vi "泰克1路.vi"() -> ()   [LabVIEW 2018]
uses:
  <instrlib>/Tektronix DPO MSO 2000 4000 Series/Public/Configure/Configure Trigger (Edge).vi
  <vilib>/Utility/file.llb/Write Delimited Spreadsheet (string).vi
  <instrlib>/Tektronix DPO MSO 2000 4000 Series/Tektronix DPO MSO 2000 4000 Series.lvlib
  <vilib>/Utility/file.llb/Write Delimited Spreadsheet (DBL).vi
panel:
  out "波形图表":waveform(dbl)(graph)
  out "Frequency":dbl
  out "rasing":dbl
  out "error out":errorcluster
  in  "停止":bool
  out "num":u32
  in  "VISA Resource Name":refnum<visa-resource-name>="TCPIP::192.168.129.100::INSTR"
  in  "VoltRange-1(V=10*grid)":dbl=0.005
  in  "Trigger Level (V)":dbl=0.01
  in  "Timebase(s)":dbl=4e-08
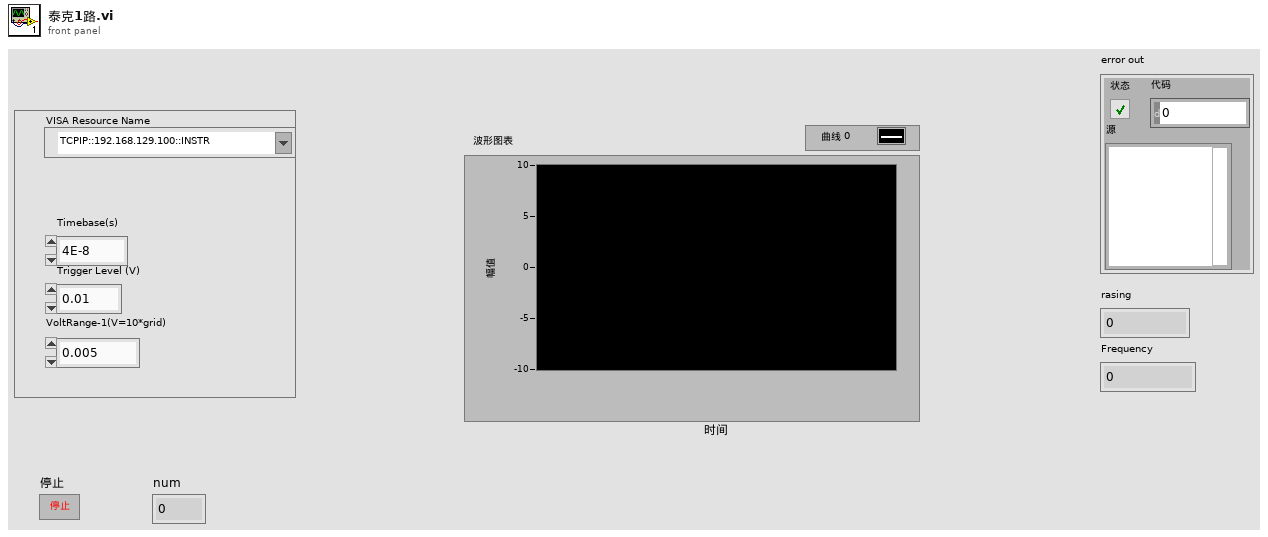
[diagram p1: front panel]
types:
  T1 = enum16{"Channel 1", "Channel 2", "Channel 3", "Channel 4", "Math", "Reference 1", "Reference 2", "Reference 3", "Reference 4"}
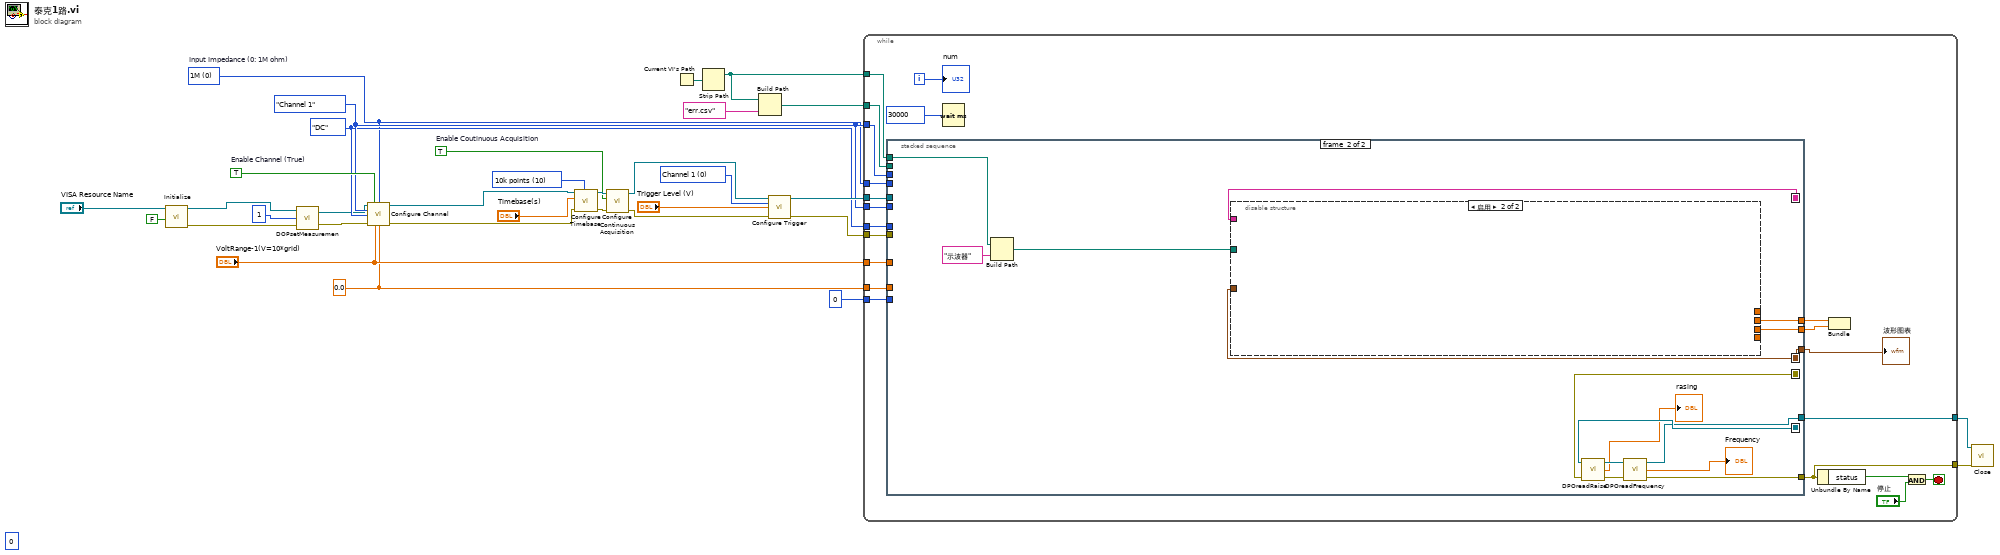
[diagram p0: block diagram]
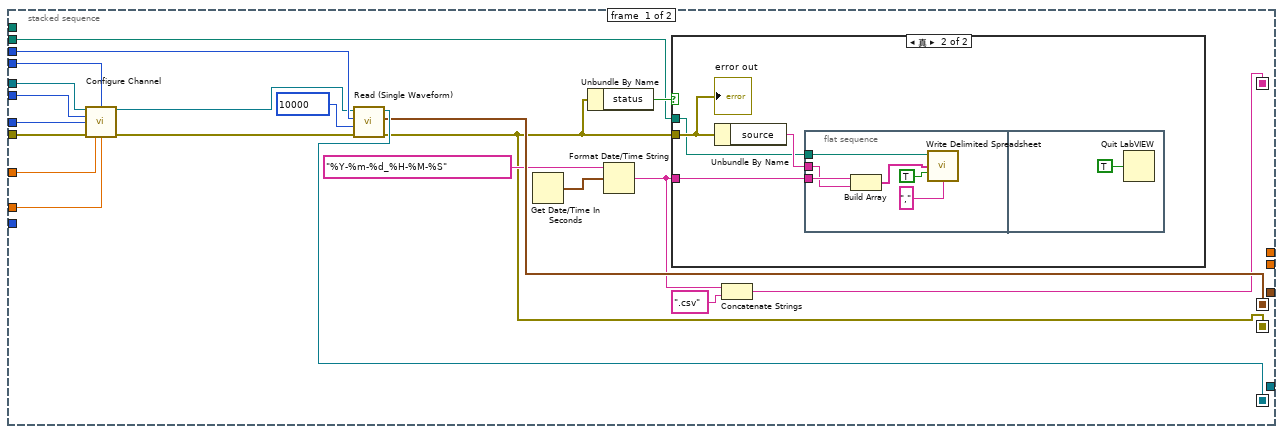
[diagram p2: hidden frame]
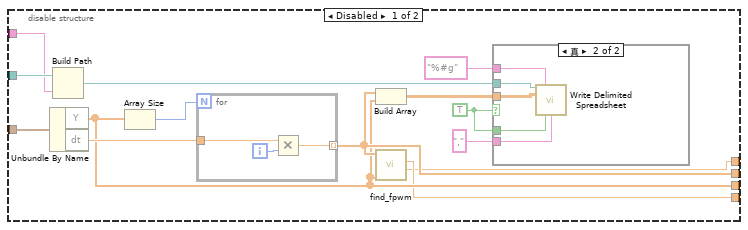
[diagram p4: hidden frame]
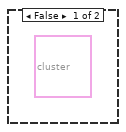
[diagram p5: hidden frame]
diagram:
  w31 = u32 10 items=["1000 points"=1, "10k points"=10, "100k points"=100, "1M points"=1000, "5M points"=5000, "10M points"=10000] ("Record Length (10: 10k points)")
  w1 = 0.0 ("VoltOffset-1(0.0V)")
  w13 = T1."Channel 1" ("Channel (0:Channel 1)")
  w12 = enum16{"AC", "DC", "Ground"}."DC" ("VoltCoupling-1&2(1:DC)")
  (unwired) 0 ("mode")
  w19 = u16 0 items=["Channel 1", "Channel 2", "Channel 3", "Channel 4", "AC Line", "Aux", "Digital Channel 0", "Digital Channel 1", "Digital Channel 2", "Digital Channel 3", "Digital Channel 4", "Digital Channel 5", "Digital Channel 6", "Digital Channel 7", "Digital Channel 8", "Digital Channel 9", "Digital Channel 10", "Digital Channel 11", "Digital Channel 12", "Digital Channel 13", "Digital Channel 14", "Digital Channel 15", "RF"] ("Trigger Source (0: Channel 1)")
  w11 = u16 0 items=["1M", "75", "50"]  # Input Impedance (0: 1M ohm)
  w21 = TRUE  # Enable Coutinuous Acquisition
  w20 = TRUE  # Enable Channel (True)
  n1 = call <instrlib>:"Initialize.vi"("Reset (True)"=FALSE, "VISA resource name"="VISA Resource Name") -> ("error out"=w6:errorcluster, "VISA resource name out"=w7:refnum<visa-resource-name>)  [unwired: 8 in]
  n2 = call "DOPsetMeasuremen.vi"("error in (no error)"=w6, "CH"=u8 1, "VISA resource name"=w7) -> ("error out"=w4:errorcluster, "VISA resource name out"=w5:refnum<visa-resource-name>)
  n3 = call <instrlib>:"Configure Channel.vi"("VISA resource name"=w5, "Enable Channel (T: Enable)"=w20, "Input Impedance (0: 1M ohm)"=w11, "Channel (0: Channel 1)"=w13, "Vertical Coupling (1: DC)"=w12, "error in (no error)"=w4, "Vertical Range (10.0 V)"="VoltRange-1(V=10*grid)", "Vertical Offset (0.0 V)"=w1) -> ("VISA resource name out"=w26:refnum<visa-resource-name>, "error out"=w23:errorcluster)  [unwired: 6 in]
  n4 = call <instrlib>:"Configure Timebase.vi"("Record Length (10: 10k points)"=w31, "error in (no error)"=w23, "Timebase (0.0005 s)"="Timebase(s)", "VISA resource name"=w26) -> ("error out"=w24:errorcluster, "VISA resource name out"=w28:refnum<visa-resource-name>)  [unwired: 6 in]
  n5 = call <instrlib>:"Configure Continuous Acquisition.vi"("error in (no error)"=w24, "Enable Continuous Acquisition Mode (T: Enable)"=w21, "VISA resource name"=w28) -> ("error out"=w25:errorcluster, "VISA resource name out"=w29:refnum<visa-resource-name>)  [unwired: 7 in]
  n6 = Current VI's Path() -> (path=w15:path)
  n7 = Strip Path(path=w15) -> (stripped path=w10:path)  [unwired: 1 out]
  n8 = Build Path(base path=w10, name or relative path="err.csv" ("名称或相对路径")) -> (appended path=w8:path)
  n9 = call-poly <instrlib>:"Configure Trigger.vi"("VISA resource name"=w29, "Trigger Source (0: Channel 1)"=w19, "Trigger Level (0.0 V)"="Trigger Level (V)", "error in (no error)"=w25) -> ("VISA resource name out"=w17:refnum<visa-resource-name>, "error out"=w16:errorcluster)  [unwired: 10 in]
  n10 = while {
    tunnel: [w54] -> w33
    tunnel: [w44] -> w32
    tunnel: w17 -> [w53]
    tunnel: w16 -> [w52]
    tunnel: w13 -> [w51]
    tunnel: w10 -> [w50]
    tunnel: 0 ("index") -> [w49]
    tunnel: w13 -> [w40]
    tunnel: w12 -> [w39]
    tunnel: "VoltRange-1(V=10*grid)" -> [w38]
    tunnel: w1 -> [w37]
    tunnel: w11 -> [w36]
    tunnel: w8 -> [w35]
    i -> [w47]
    stop <- w41 stop-if-true
    n11 = stacked-sequence {
      seq-local: [w75 _] -> [_ w95]
      seq-local: [w57 _] -> [_ w92]
      seq-local: [w73 _] -> [_ w89]
      seq-local: [w69 _] -> [_ w98]
      tunnel: w53 -> [w67 _]
      tunnel: w52 -> [w65 _]
      tunnel: w51 -> [w74 _]
      tunnel: [_ w93] -> w54
      tunnel: [_ w90] -> w44
      tunnel: w50 -> [_ w101]
      tunnel: w49 -> [_ _]
      tunnel: [_ w97] -> w46
      tunnel: [_ w96] -> w45
      tunnel: w40 -> [w63 _]
      tunnel: w39 -> [w62 _]
      tunnel: w38 -> [w61 _]
      tunnel: w37 -> [w60 _]
      tunnel: w36 -> [w59 _]
      tunnel: w35 -> [w56 _]
      tunnel: [_ w89] -> w34
      frame #0 {
        n12 = call <instrlib>:"Configure Channel.vi"("VISA resource name"=w67, "Input Impedance (0: 1M ohm)"=w59, "Channel (0: Channel 1)"=w63, "Vertical Coupling (1: DC)"=w62, "error in (no error)"=w65, "Vertical Range (10.0 V)"=w61, "Vertical Offset (0.0 V)"=w60) -> ("VISA resource name out"=w66:refnum<visa-resource-name>, "error out"=w64:errorcluster)  [unwired: 7 in]
        n13 = call <instrlib>:"Read (Single Waveform).vi"("error in (no error)"=w64, "Maximum Time (10000ms)"=u32 10000 ("Maximum Time(10000ms)"), "Channel (0: Channel 1)"=w74, "VISA resource name"=w66) -> ("error out"=w57:errorcluster, "Waveform Graph"=w73:waveform(dbl), "VISA resource name out"=w75:refnum<visa-resource-name>)  [unwired: 5 in]
        n14 = Get Date/Time In Seconds() -> (seconds since 1Jan1904=w71:timestamp)
        n15 = Unbundle By Name(w57) -> ("status"=w58:bool)
        n16 = Format Date/Time String(time format string (%c)="%Y-%m-%d_%H-%M-%S" ("时间格式字符串(%c)"), seconds (now)=w71) -> (date/time string=w55:string)  [unwired: 1 in]
        n17 = case shown="真" w58 {
          tunnel: w57 -> [_ w79]
          tunnel: w56 -> [_ w76]
          tunnel: w55 -> [_ w77]
          frame False {
          }
          frame True {
            n18 = Unbundle By Name(w79) -> ("source"=w78:string)
            n19 = flat-sequence {
              tunnel: w78 -> [w84]
              tunnel: w77 -> [w85]
              tunnel: w76 -> [w82]
              frame #0 {
                n20 = Build Array(w85, w84) -> (w83:string[])
                n21 = call-poly <vilib>:"Write Delimited Spreadsheet.vi"("file path (dialog if empty)"=w82, "1D data"=w83, "append to file? (new file:F)"=TRUE, "delimiter (\\t)"="," ("delimiter (\\t)")) -> ()  [unwired: 10 in, 2 out]
              }
              frame #1 {
                n22 = Quit LabVIEW(quit? (T)=TRUE) -> ()
              }
            }
            "error out" <- w79
          }
        }
        n23 = Concatenate Strings(w55, ".csv" ("字符串")) -> (w69:string)
      }
      frame #1 {
        n24 = Build Path(base path=w101, name or relative path="示波器" ("名称或相对路径")) -> (appended path=w99:path)
        n25 = disable-structure shown="启用" {
          disable-tunnel: w99 -> [w115 _]
          disable-tunnel: w98 -> [w114 _]
          disable-tunnel: w89 -> [w111 _]
          disable-tunnel: [w105 _] -> w97
          disable-tunnel: [w104 _] -> w96
          disable-tunnel: [w103 _] -> _
          disable-tunnel: [w102 _] -> _
          frame Disabled {
            w106 = TRUE ("transpose? (no:F)")
            n26 = Unbundle By Name(w111) -> ("Y"=w104:dbl[], "dt"=w110:dbl)
            n27 = Build Path(base path=w115, name or relative path=w114) -> (appended path=w113:path)
            n28 = Array Size(array=w104) -> (size(s)=w108:i32)
            n29 = for {
              N: w108 -> [_]
              tunnel: w110 -> [w118]
              tunnel: [w116] -> w105 mode=indexing
              i -> [w117]
              n30 = Multiply(x=w118, y=w117) -> (x*y=w116:dbl)
            }
            n31 = Build Array(w105, w104) -> (w109:dbl[][])
            n32 = call "find_fpwm.vi"("Y"=w104, "X"=w105) -> ("FPWM"=w102:dbl, "rasing"=w103:dbl)  [unwired: 5 in, 3 out]
            n33 = case shown="真" w106 {
              tunnel: w113 -> [_ w124]
              tunnel: "," ("delimiter (\\t)") -> [_ w123]
              tunnel: w109 -> [_ w122]
              tunnel: w106 -> [_ w121]
              tunnel: "%#g" ("format (%.3f)") -> [_ w120]
              frame False {
                w119 = cluster{dbl[], dbl[]} {array[100000 elements], array[100000 elements]}
              }
              frame True {
                n34 = call-poly <vilib>:"Write Delimited Spreadsheet.vi"("file path (dialog if empty)"=w124, "format (%.3f)"=w120, "2D data"=w122, "transpose? (no:F)"=w121, "delimiter (\\t)"=w123) -> ()  [unwired: 9 in, 2 out]
              }
            }
          }
          frame Enabled {
          }
        }
        n35 = call "DPOreadRaise.vi"("错误输入（无错误）"=w92, "VISA资源名称"=w95) -> ("错误输出"=w91:errorcluster, "上升沿时间"=→"rasing":dbl, "VISA资源名称输出"=w94:refnum<visa-resource-name>)  [unwired: 1 in]
        n36 = call "DPOreadFrequency.vi"("错误输入（无错误）"=w91, "VISA资源名称"=w94) -> ("错误输出"=w90:errorcluster, "重复频率"=→"Frequency":dbl, "VISA资源名称输出"=w93:refnum<visa-resource-name>)  [unwired: 1 in]
      }
    }
    "波形图表" <- w34
    n37 = Wait (ms)(milliseconds to wait=u32 30000 ("等待时间（毫秒）")) -> ()  [unwired: 1 out]
    n38 = Unbundle By Name(w44) -> ("status"=w43:bool)
    n39 = Bundle(w46, "Y"=w45) -> ()  [unwired: 1 in, 1 out]
    n40 = And(x=w43, y="停止") -> (x .and. y?=w41:bool)
    "num" <- w47
  }
  n41 = call <instrlib>:"Close.vi"("error in (no error)"=w32, "VISA resource name"=w33) -> ()  [unwired: 9 in, 1 out]
